vi "List Directory__ogtk.vi"(4 "error in (no error)":errorcluster, 6 "pattern":string, 7 "directory path":path) -> (0 "error out":errorcluster, 1 "directory names":string[](array[string]), 2 "file names":string[](array[string]), 3 "dup directory path":path)   [LabVIEW 2014]
doc: "Augments the primitive List Directory function by allowing multiple semicolon delimited patterns."
uses:
  <userlib>/_OpenG.lib/string/string.llb/Trim Whitespace (String)__ogtk.vi
  <userlib>/_OpenG.lib/array/array.llb/Remove Duplicates from 1D Array (String)__ogtk.vi
panel:
  # "List Directory.vi\n\nAugments the primitive List Directory function by\nallowing semicolon delimited patterns.\n\nPlease visit http://www.OpenG.org to learn about the\nOpen Source LabVIEW software movement.\n\nNOTICE -- YOU MUST LEAVE THIS NOTICE IN PLACE.  PER THE TERMS OF THE LICENSE BELOW, YOU MAY SUBLICENSE THIS SOFTWARE \nIN ANY WAY THAT DOES NOT CONFLICT WITH THIS LICENSE.\n\n### BSD License (http://www.opensource.org/licenses/bsd-license.php) Begin ###\n \nCopyright (c) 2002-2006, Jim Kring <jim@jimkring.com>\n\nAll rights reserved.\n\nRedistribution and use in source and binary forms, with or without modification, are permitted provided that the following conditions are met:\n\n    * Redistributions of source code must retain the above copyright notice, this list of conditions and the following disclaimer.\n    * Redistributions in binary form must reproduce the above copyright notice, this list of conditions and the following disclaimer in the \n       documentation and/or other materials provided with the distribution.\n    * Neither the name of SciWare, James Kring, Inc., nor the names of its contributors may be used to endorse or promote products derived \n       from this software without specific prior written permission.\n\nTHIS SOFTWARE IS PROVIDED BY THE COPYRIGHT HOLDERS AND CONTRIBUTORS \"AS IS\" AND ANY EXPRESS OR IMPLIED WARRANTIES, \nINCLUDING, BUT NOT LIMITED TO, THE IMPLIED WARRANTIES OF MERCHANTABILITY AND FITNESS FOR A PARTICULAR PURPOSE ARE \nDISCLAIMED. IN NO EVENT SHALL THE COPYRIGHT OWNER OR CONTRIBUTORS BE LIABLE FOR ANY DIRECT, INDIRECT, INCIDENTAL,\n SPECIAL, EXEMPLARY, OR CONSEQUENTIAL DAMAGES (INCLUDING, BUT NOT LIMITED TO, PROCUREMENT OF SUBSTITUTE GOODS OR \nSERVICES; LOSS OF USE, DATA, OR PROFITS; OR BUSINESS INTERRUPTION) HOWEVER CAUSED AND ON ANY THEORY OF LIABILITY, \nWHETHER IN CONTRACT, STRICT LIABILITY, OR TORT (INCLUDING NEGLIGENCE OR OTHERWISE) ARISING IN ANY WAY OUT OF THE USE \nOF THIS SOFTWARE, EVEN IF ADVISED OF THE POSSIBILITY OF SUCH DAMAGE.\n\n### BSD License End ###"
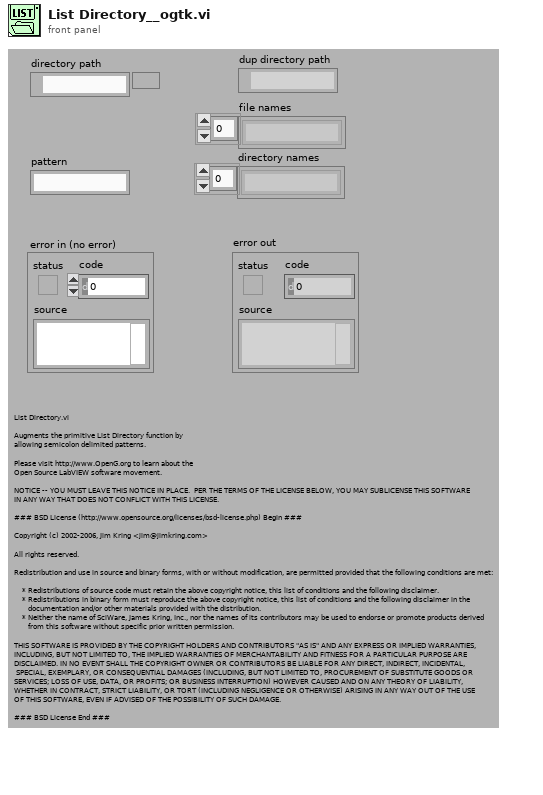
[diagram p1: front panel]
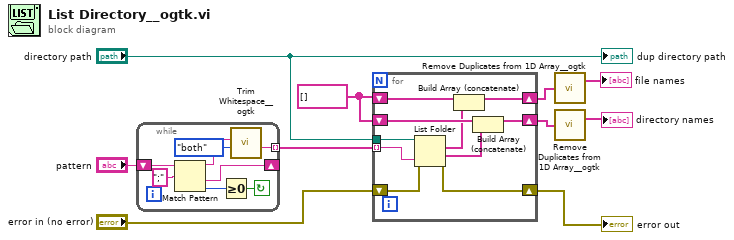
[diagram p0: block diagram]
diagram:
  w5 = string[] [] ("file names")
  n1 = while {
    shift-right: [w18] -> _
    shift-left: "pattern" -> [w15]
    tunnel: [w12] -> w10 mode=indexing
    stop <- w17 continue-if-true
    n2 = Match Pattern(string=w15, regular expression=";" ("pattern")) -> (before substring=w14:string, after substring=w18:string, offset past match=w16:i32)  [unwired: 1 in, 1 out]
    n3 = Greater Or Equal To 0?(x=w16) -> (x >= 0?=w17:bool)
    n4 = call-poly <userlib>:"Trim Whitespace__ogtk.vi"("Remove (leading and trailing)"=enum16{"leading", "trailing", "both"}."both" ("remove (leading and trailing)"), "String in"=w14) -> ("String out"=w12:string)  [unwired: 5 in]
  }
  n5 = for {
    tunnel: w10 -> [w28] mode=indexing
    shift-right: [w26] -> w8
    shift-left: "error in (no error)" -> [w27]
    tunnel: "directory path" -> [w25]
    shift-right: [w23] -> w2
    shift-left: w5 -> [w24]
    shift-right: [w21] -> w4
    shift-left: w5 -> [w22]
    n6 = List Folder(path=w25, pattern=w28, error in=w27) -> (filenames=w19:string[], folder names=w20:string[], error out=w26:errorcluster)  [unwired: 1 in, 1 out]
    n7 = Build Array (concatenate)(w24, w19) -> (w23:string[])
    n8 = Build Array (concatenate)(w22, w20) -> (w21:string[])
  }
  "error out" <- w8
  n9 = call-poly <userlib>:"Remove Duplicates from 1D Array__ogtk.vi"("Input Array"=w2) -> ("Output Array"=→"file names":string[])  [unwired: 1 out]
  n10 = call-poly <userlib>:"Remove Duplicates from 1D Array__ogtk.vi"("Input Array"=w4) -> ("Output Array"=→"directory names":string[])  [unwired: 1 out]
  "dup directory path" <- "directory path"
